vi "Query Waveform Shape.vi"(8 "error in (no error)":errorcluster, 10 "Channel (0: Channel 1)":T2 items=["Channel 1", "Channel 2"], 11 "VISA resource name":refnum<visa-resource-name>) -> (0 "error out":errorcluster, 1 "Waveform Shape":T1 items=["Sinusoid", "Square", "Pulse", "Ramp", "PRNoise", "DC", "SINC", "Gaussian", "Lorentz", "ERise", "EDecay", "Haversine", "User 1", "User 2", "User 3", "User 4", "EMemory", "EFile"], 3 "VISA resource name out":refnum<visa-resource-name>)   [LabVIEW 2009, in "Tektronix AFG 3000 Series.lvlib"]
doc: "Queries the shape of the output waveform on a Tektronix AFG 3000 series function generator."
uses:
  Tektronix AFG 3000 Series.lvlib
  controls.llb/Channel.ctl
  controls.llb/Waveform Shape.ctl
  <vilib>/Utility/error.llb/DialogType.ctl
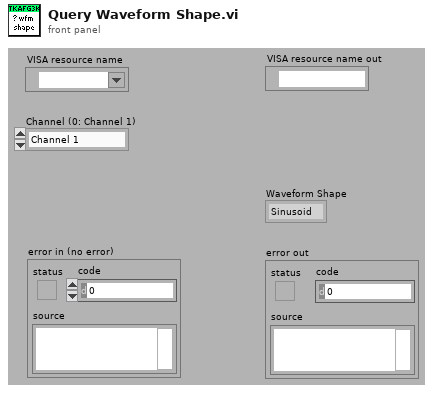
[diagram p1: front panel]
types:
  T1 = typedef "Waveform Shape.ctl" = u16
  T2 = typedef "Channel.ctl" = u16
  T3 = typedef "DialogType.ctl" = u16
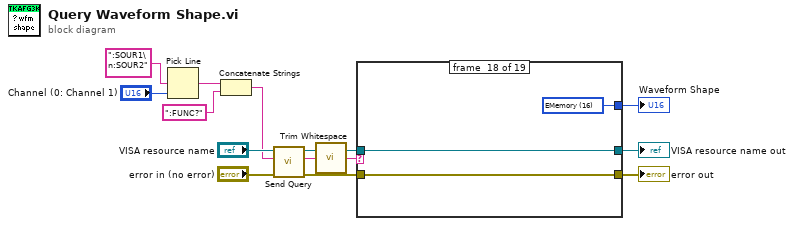
[diagram p0: block diagram]
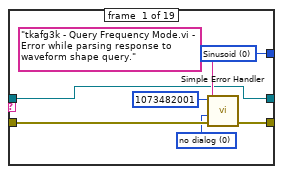
[diagram p2: hidden frame]
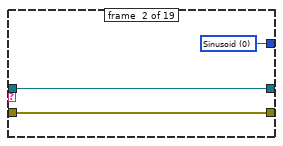
[diagram p3: hidden frame]
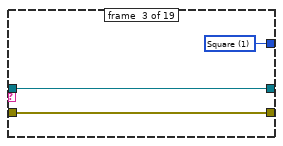
[diagram p4: hidden frame]
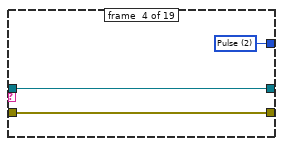
[diagram p5: hidden frame]
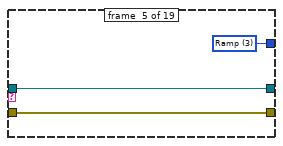
[diagram p6: hidden frame]
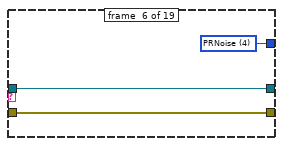
[diagram p7: hidden frame]
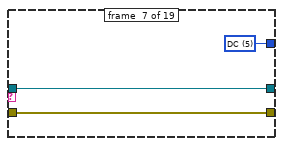
[diagram p8: hidden frame]
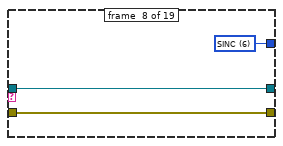
[diagram p9: hidden frame]
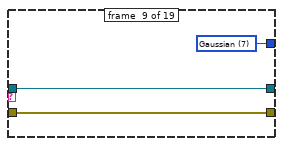
[diagram p10: hidden frame]
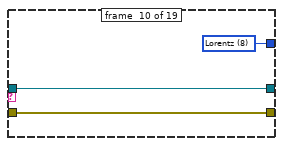
[diagram p11: hidden frame]
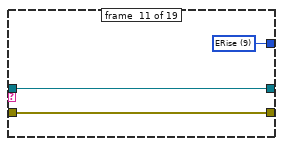
[diagram p12: hidden frame]
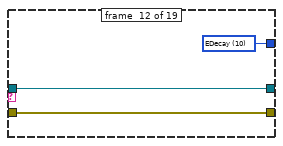
[diagram p13: hidden frame]
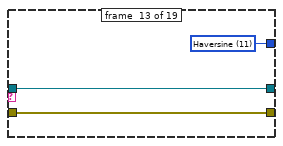
[diagram p14: hidden frame]
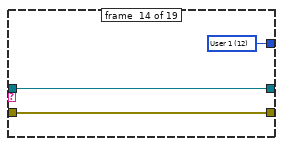
[diagram p15: hidden frame]
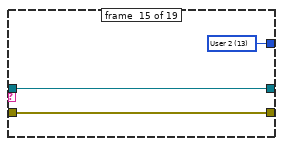
[diagram p16: hidden frame]
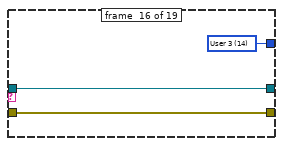
[diagram p17: hidden frame]
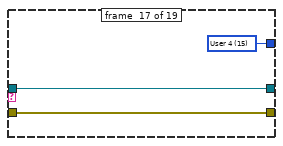
[diagram p18: hidden frame]
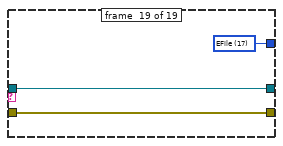
[diagram p19: hidden frame]
diagram:
  n1 = Pick Line(multi-line string=":SOUR1\n:SOUR2", line index="Channel (0: Channel 1)") -> (output string=w11:string)  [unwired: 1 out]
  n2 = Concatenate Strings(w11, ":FUNC?" ("format string")) -> (w10:string)
  n3 = call "Send Query.vi"("error in (no error)"="error in (no error)", "write buffer"=w10, "VISA resource name"="VISA resource name") -> ("error out"=w7:errorcluster, "read buffer"=w3:string, "VISA resource name out"=w6:refnum<visa-resource-name>)  [unwired: 1 in, 5 out]
  n4 = call <vilib>:"Trim Whitespace.vi"("string"=w3) -> ("trimmed string"=w2:string)  [unwired: 1 in]
  n5 = case shown="Default" w2 {
    tunnel: [w15 w22 w25 w28 w31 w34 w37 w40 w43 w46 w49 w52 w55 w58 w61 w64 w67 w70 w73] -> w1
    tunnel: w7 -> [w21 w23 w26 w29 w32 w35 w38 w41 w44 w47 w50 w53 w56 w59 w62 w65 w68 w71 w74]
    tunnel: w6 -> [w16 w24 w27 w30 w33 w36 w39 w42 w45 w48 w51 w54 w57 w60 w63 w66 w69 w72 w75]
    tunnel: [w16 w24 w27 w30 w33 w36 w39 w42 w45 w48 w51 w54 w57 w60 w63 w66 w69 w72 w75] -> w5
    tunnel: [w20 w23 w26 w29 w32 w35 w38 w41 w44 w47 w50 w53 w56 w59 w62 w65 w68 w71 w74] -> w4
    frame #0 {
      w15 = T1 0 items=["Sinusoid", "Square", "Pulse", "Ramp", "PRNoise", "DC", "SINC", "Gaussian", "Lorentz", "ERise", "EDecay", "Haversine", "User 1", "User 2", "User 3", "User 4", "EMemory", "EFile"] ("Waveform Shape 2")
      w19 = T3 0 items=["no dialog", "OK message", "continue or stop message", "OK message + warnings", "continue/stop + warnings"] ("type of dialog (OK msg:1)")
      n6 = call <vilib>:"Simple Error Handler.vi"("error code (no error:0)"=1073482001, "error source (\" \")"="tkafg3k - Query Frequency Mode.vi - Error while parsing response to waveform shape query." ("error source (\" \")"), "type of dialog (OK msg:1)"=w19, "error in (no error)"=w21) -> ("error out"=w20:errorcluster)  [unwired: 5 out]
    }
    frame #1 {
      w22 = T1 0 items=["Sinusoid", "Square", "Pulse", "Ramp", "PRNoise", "DC", "SINC", "Gaussian", "Lorentz", "ERise", "EDecay", "Haversine", "User 1", "User 2", "User 3", "User 4", "EMemory", "EFile"] ("Waveform Shape 2")
    }
    frame #2 {
      w25 = T1 1 items=["Sinusoid", "Square", "Pulse", "Ramp", "PRNoise", "DC", "SINC", "Gaussian", "Lorentz", "ERise", "EDecay", "Haversine", "User 1", "User 2", "User 3", "User 4", "EMemory", "EFile"] ("Waveform Shape 2")
    }
    frame #3 {
      w28 = T1 2 items=["Sinusoid", "Square", "Pulse", "Ramp", "PRNoise", "DC", "SINC", "Gaussian", "Lorentz", "ERise", "EDecay", "Haversine", "User 1", "User 2", "User 3", "User 4", "EMemory", "EFile"] ("Waveform Shape 2")
    }
    frame #4 {
      w31 = T1 3 items=["Sinusoid", "Square", "Pulse", "Ramp", "PRNoise", "DC", "SINC", "Gaussian", "Lorentz", "ERise", "EDecay", "Haversine", "User 1", "User 2", "User 3", "User 4", "EMemory", "EFile"] ("Waveform Shape 2")
    }
    frame #5 {
      w34 = T1 4 items=["Sinusoid", "Square", "Pulse", "Ramp", "PRNoise", "DC", "SINC", "Gaussian", "Lorentz", "ERise", "EDecay", "Haversine", "User 1", "User 2", "User 3", "User 4", "EMemory", "EFile"] ("Waveform Shape 2")
    }
    frame #6 {
      w37 = T1 5 items=["Sinusoid", "Square", "Pulse", "Ramp", "PRNoise", "DC", "SINC", "Gaussian", "Lorentz", "ERise", "EDecay", "Haversine", "User 1", "User 2", "User 3", "User 4", "EMemory", "EFile"] ("Waveform Shape 2")
    }
    frame #7 {
      w40 = T1 6 items=["Sinusoid", "Square", "Pulse", "Ramp", "PRNoise", "DC", "SINC", "Gaussian", "Lorentz", "ERise", "EDecay", "Haversine", "User 1", "User 2", "User 3", "User 4", "EMemory", "EFile"] ("Waveform Shape 2")
    }
    frame #8 {
      w43 = T1 7 items=["Sinusoid", "Square", "Pulse", "Ramp", "PRNoise", "DC", "SINC", "Gaussian", "Lorentz", "ERise", "EDecay", "Haversine", "User 1", "User 2", "User 3", "User 4", "EMemory", "EFile"] ("Waveform Shape 2")
    }
    frame #9 {
      w46 = T1 8 items=["Sinusoid", "Square", "Pulse", "Ramp", "PRNoise", "DC", "SINC", "Gaussian", "Lorentz", "ERise", "EDecay", "Haversine", "User 1", "User 2", "User 3", "User 4", "EMemory", "EFile"] ("Waveform Shape 2")
    }
    frame #10 {
      w49 = T1 9 items=["Sinusoid", "Square", "Pulse", "Ramp", "PRNoise", "DC", "SINC", "Gaussian", "Lorentz", "ERise", "EDecay", "Haversine", "User 1", "User 2", "User 3", "User 4", "EMemory", "EFile"] ("Waveform Shape 2")
    }
    frame #11 {
      w52 = T1 10 items=["Sinusoid", "Square", "Pulse", "Ramp", "PRNoise", "DC", "SINC", "Gaussian", "Lorentz", "ERise", "EDecay", "Haversine", "User 1", "User 2", "User 3", "User 4", "EMemory", "EFile"] ("Waveform Shape 2")
    }
    frame #12 {
      w55 = T1 11 items=["Sinusoid", "Square", "Pulse", "Ramp", "PRNoise", "DC", "SINC", "Gaussian", "Lorentz", "ERise", "EDecay", "Haversine", "User 1", "User 2", "User 3", "User 4", "EMemory", "EFile"] ("Waveform Shape 2")
    }
    frame #13 {
      w58 = T1 12 items=["Sinusoid", "Square", "Pulse", "Ramp", "PRNoise", "DC", "SINC", "Gaussian", "Lorentz", "ERise", "EDecay", "Haversine", "User 1", "User 2", "User 3", "User 4", "EMemory", "EFile"] ("Waveform Shape 2")
    }
    frame #14 {
      w61 = T1 13 items=["Sinusoid", "Square", "Pulse", "Ramp", "PRNoise", "DC", "SINC", "Gaussian", "Lorentz", "ERise", "EDecay", "Haversine", "User 1", "User 2", "User 3", "User 4", "EMemory", "EFile"] ("Waveform Shape 2")
    }
    frame #15 {
      w64 = T1 14 items=["Sinusoid", "Square", "Pulse", "Ramp", "PRNoise", "DC", "SINC", "Gaussian", "Lorentz", "ERise", "EDecay", "Haversine", "User 1", "User 2", "User 3", "User 4", "EMemory", "EFile"] ("Waveform Shape 2")
    }
    frame #16 {
      w67 = T1 15 items=["Sinusoid", "Square", "Pulse", "Ramp", "PRNoise", "DC", "SINC", "Gaussian", "Lorentz", "ERise", "EDecay", "Haversine", "User 1", "User 2", "User 3", "User 4", "EMemory", "EFile"] ("Waveform Shape 2")
    }
    frame #17 {
      w70 = T1 16 items=["Sinusoid", "Square", "Pulse", "Ramp", "PRNoise", "DC", "SINC", "Gaussian", "Lorentz", "ERise", "EDecay", "Haversine", "User 1", "User 2", "User 3", "User 4", "EMemory", "EFile"] ("Waveform Shape 2")
    }
    frame #18 {
      w73 = T1 17 items=["Sinusoid", "Square", "Pulse", "Ramp", "PRNoise", "DC", "SINC", "Gaussian", "Lorentz", "ERise", "EDecay", "Haversine", "User 1", "User 2", "User 3", "User 4", "EMemory", "EFile"] ("Waveform Shape 2")
    }
  }
  "error out" <- w4
  "VISA resource name out" <- w5
  "Waveform Shape" <- w1
